vi "Configure Steps.vi"(8 "error in (no error)":errorcluster, 11 "Servo MSMT in":refnum<class "Servo MSMT.lvclass">) -> (0 "error out":errorcluster, 3 "Servo MSMT out":refnum<class "Servo MSMT.lvclass">)   [LabVIEW 2018, in "Servo MSMT.lvlib" / "Servo MSMT.lvclass"]
uses:
  Servo MSMT.lvclass
  Plugins/String Database.lvlibp/String Database.lvclass
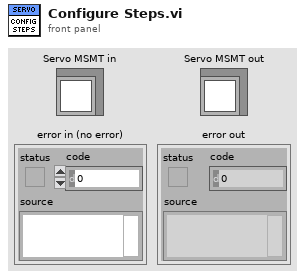
[diagram p1: front panel]
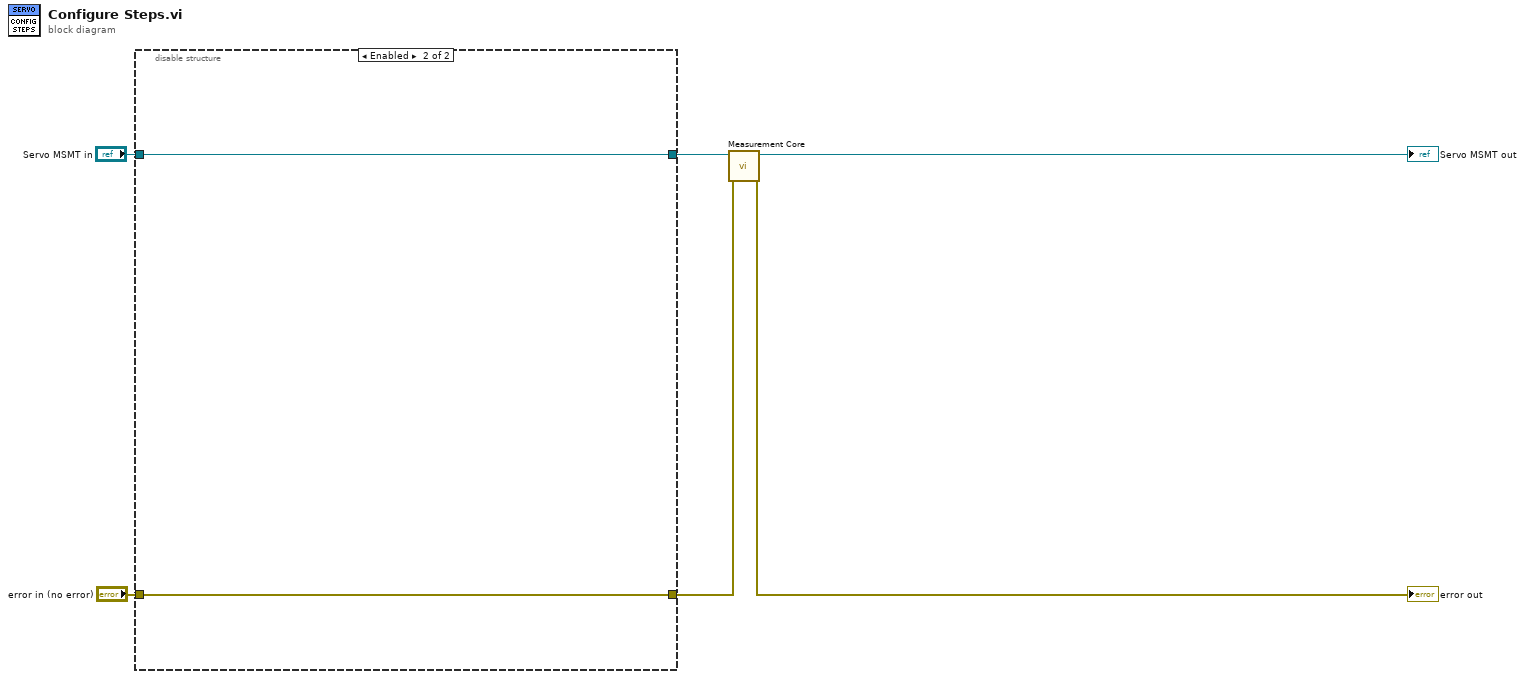
[diagram p0: block diagram]
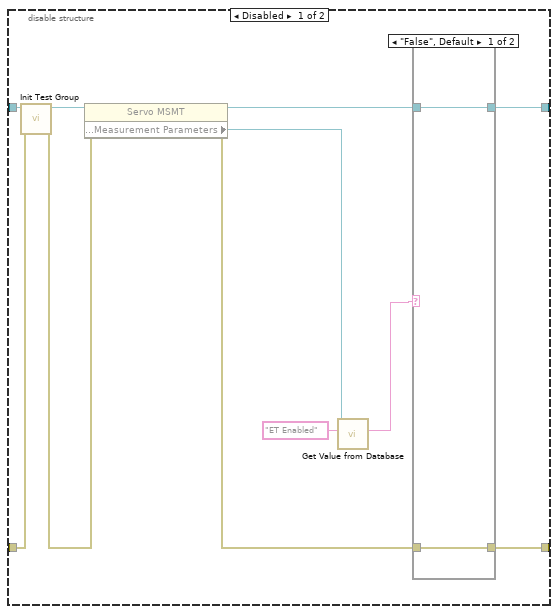
[diagram p2: hidden frame]
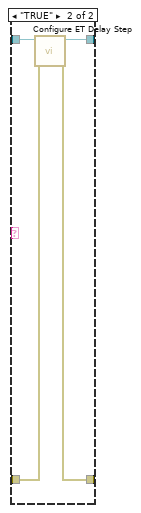
[diagram p3: hidden frame]
diagram:
  n1 = disable-structure shown="Enabled" {
    disable-tunnel: "error in (no error)" -> [w17 w24]
    disable-tunnel: [w16 w25] -> w3
    disable-tunnel: [w15 w24] -> w2
    disable-tunnel: "Servo MSMT in" -> [w7 w25]
    frame Disabled {
      n2 = call "Init Test Group.vi"("error in (no error)"=w17, "Servo MSMT in"=w7) -> ("error out"=w9:errorcluster, "Servo MSMT out"=w8:refnum<class "Servo MSMT.lvclass">)  [unwired: 8 in]
      n3 = property class="Servo MSMT"(reference=w8, error in=w9) -> (reference out=w13:refnum<class "Servo MSMT.lvclass">, error out=w14:errorcluster, "Protected Methods:Measurement Parameters"=w12:refnum<class "String Database.lvclass">)
      n4 = call "Get Value from Database.vi"("Entry Name"="ET Enabled", "Message in"=w12) -> ("Entry Value"=w10:string)  [unwired: 6 in, 3 out]
      n5 = case shown="\"False\", Default" w10 {
        tunnel: [w18 w23] -> w15
        tunnel: [w19 w22] -> w16
        tunnel: w14 -> [w18 w21]
        tunnel: w13 -> [w19 w20]
        frame "False", Default {
        }
        frame "TRUE" {
          n6 = call "Configure ET Delay Step.vi"("error in (no error)"=w21, "Servo MSMT in"=w20) -> ("error out"=w23:errorcluster, "Servo MSMT out"=w22:refnum<class "Servo MSMT.lvclass">)  [unwired: 8 in]
        }
      }
    }
    frame Enabled {
    }
  }
  n7 = call "Measurement Core.vi"("error in (no error)"=w2, "Servo MSMT in"=w3) -> ("error out"=→"error out":errorcluster, "Servo MSMT out"=→"Servo MSMT out":refnum<class "Servo MSMT.lvclass">)  [unwired: 8 in]
